vi "Write Auto Fault Recovery.vi"(8 "error in (no error)":errorcluster, 10 "Auto Fault Recovery":bool, 11 "Universal Robot in":refnum<class "Universal Robot.lvclass">) -> (0 "error out":errorcluster, 3 "Universal Robot out":refnum<class "Universal Robot.lvclass">)   [LabVIEW 2019, in "Universal Robot.lvclass"]
uses:
  Universal Robot.lvclass
  Universal Robot.lvclass/Universal Robot.ctl
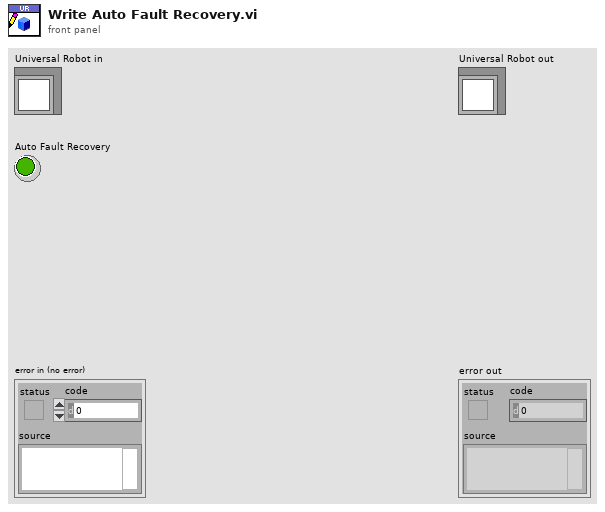
[diagram p1: front panel]
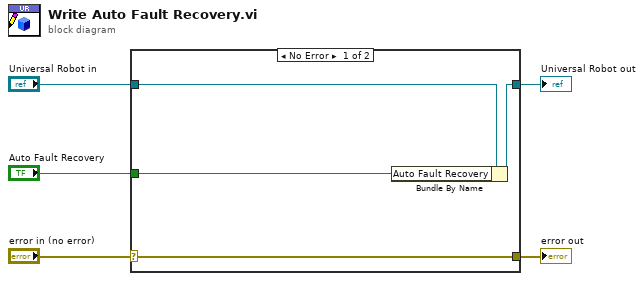
[diagram p0: block diagram]
diagram:
  n1 = case shown="No Error" "error in (no error)" {
    selector: "error in (no error)" -> [w9 w10]
    tunnel: [w9 w10] -> w4
    tunnel: [w7 w11] -> w2
    tunnel: "Universal Robot in" -> [w8 w11]
    tunnel: "Auto Fault Recovery" -> [w6 _]
    frame No Error {
      n2 = Bundle By Name(cluster=w8, "Auto Fault Recovery"=w6) -> (w7:refnum<class "Universal Robot.lvclass">)
    }
    frame Error {
    }
  }
  "error out" <- w4
  "Universal Robot out" <- w2
